vi "StomachModel.vi"() -> ()   [LabVIEW 2017]
panel:
  in  "stop":bool
  out "Ring 4 Start":u32
  out "Ring 7 Start":u32
  out "Ring 6 Start":u32
  out "Ring 5 Start":u32
  out "Ring 3 Start":u32
  out "Ring 2 Start":u32
  out "Ring 1 Start":u32
  out "Ring 0 Start":u32
  out "Run Time":u32
  in  "Time Delay 2":u32
  in  "Time Delay 1":u32
  in  "Time Delay 0":u32
  out "Ring 7":bool
  out "Ring 6":bool
  out "Ring 5":bool
  out "Ring 4":bool
  out "Ring 3":bool
  out "Ring 2":bool
  out "Ring 1":bool
  out "Time":u32
  in  "Slow Wave Generator":bool
  out "Ring 0":bool
  # "Pacemaker"
  # "Stomach Model"
  # "Ring 0"
  # "Ring 1"
  # "Ring 2"
  # "Ring 3"
  # "Ring 4"
  # "Ring 5"
  # "Corpus"
  # "Ring 6"
  # "Ring 7"
  # "Antrum"
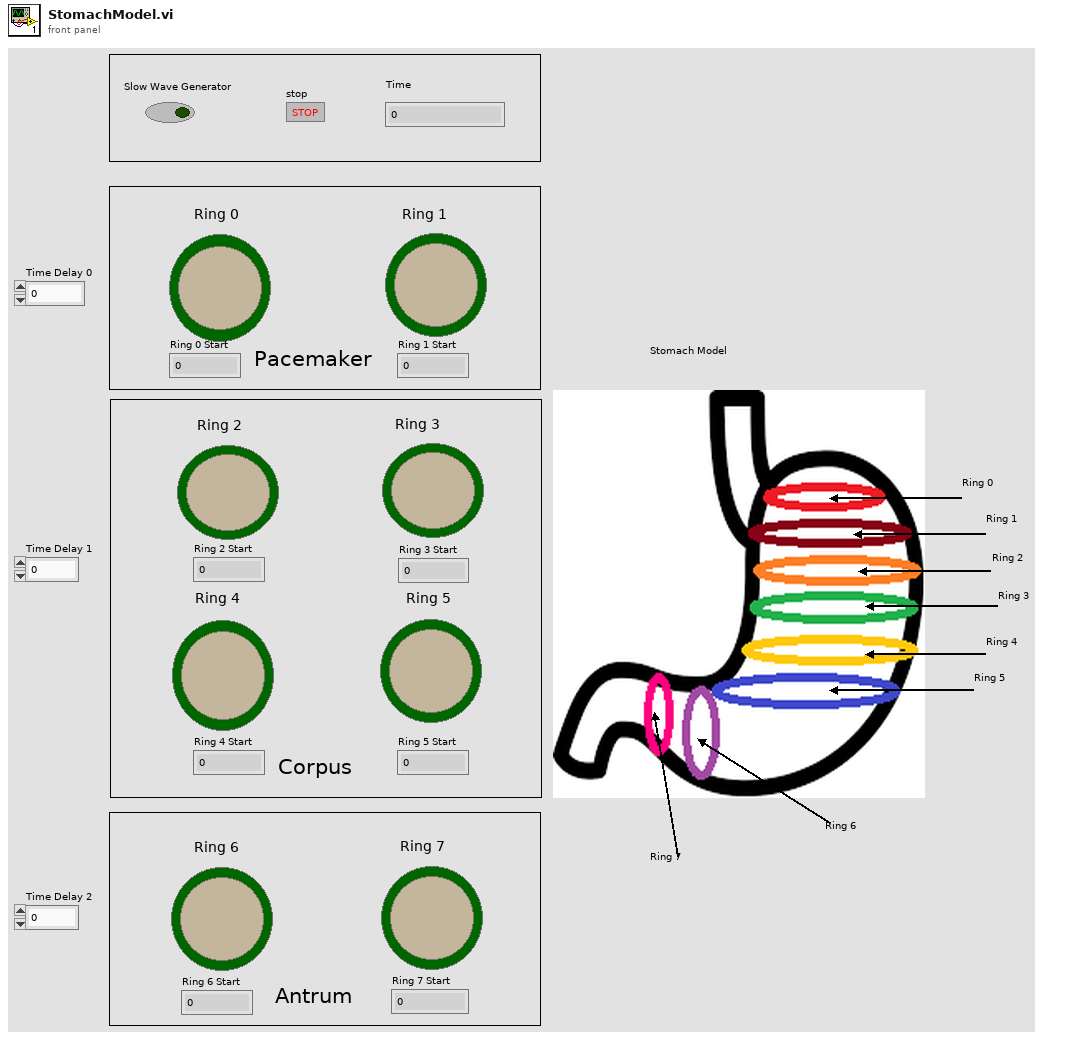
[diagram p1: front panel]
types:
  T1 = enum16{"Ring 0", "Ring 1", "Ring 2", "Ring 3", "Ring 4", "Ring 5", "Ring 6", "Ring 7"}
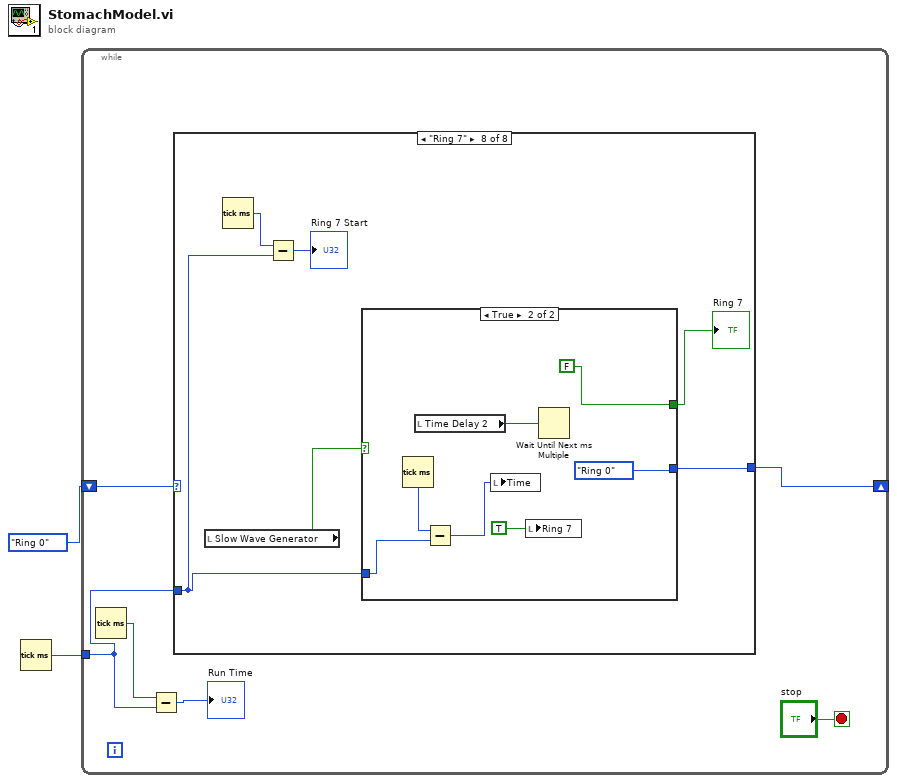
[diagram p0: block diagram]
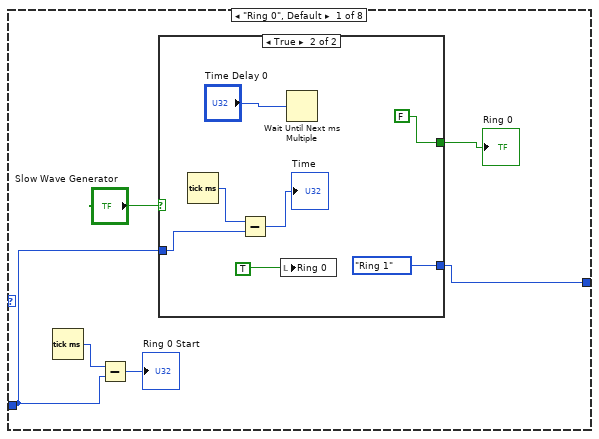
[diagram p2: hidden frame]
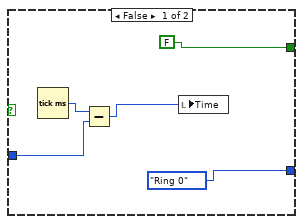
[diagram p3: hidden frame]
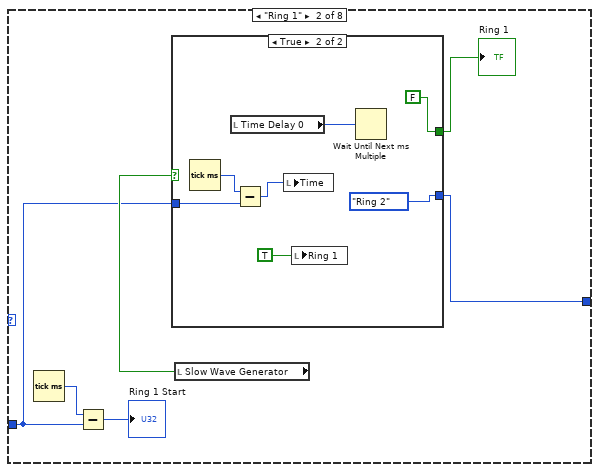
[diagram p4: hidden frame]
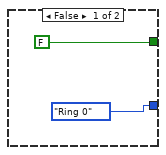
[diagram p5: hidden frame]
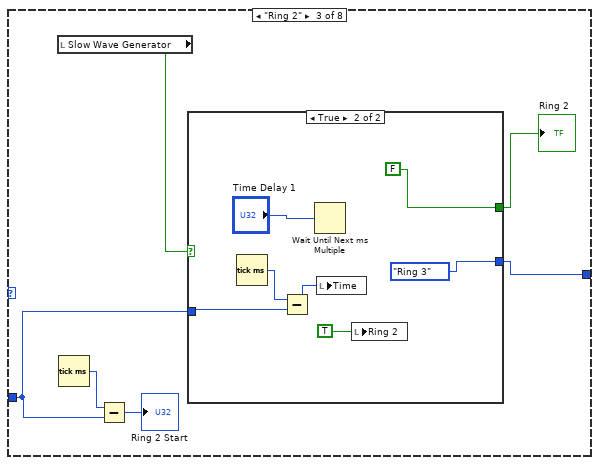
[diagram p6: hidden frame]
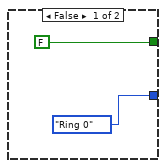
[diagram p7: hidden frame]
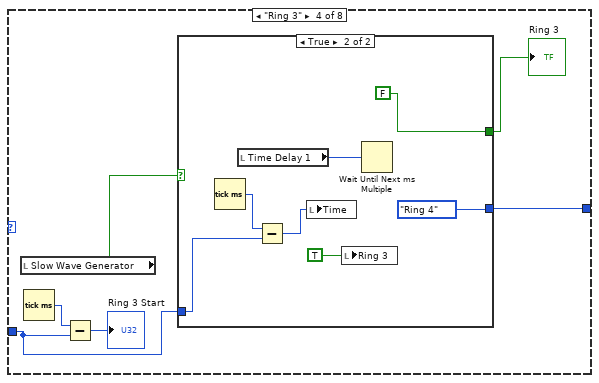
[diagram p8: hidden frame]
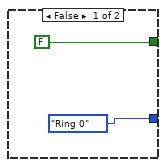
[diagram p9: hidden frame]
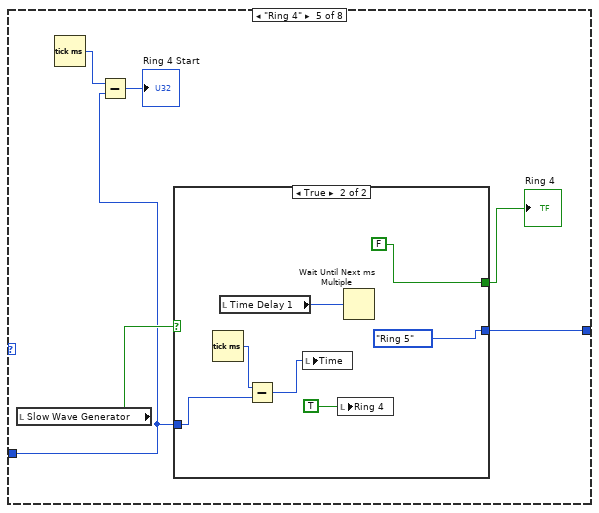
[diagram p10: hidden frame]
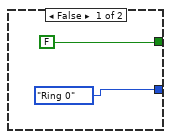
[diagram p11: hidden frame]
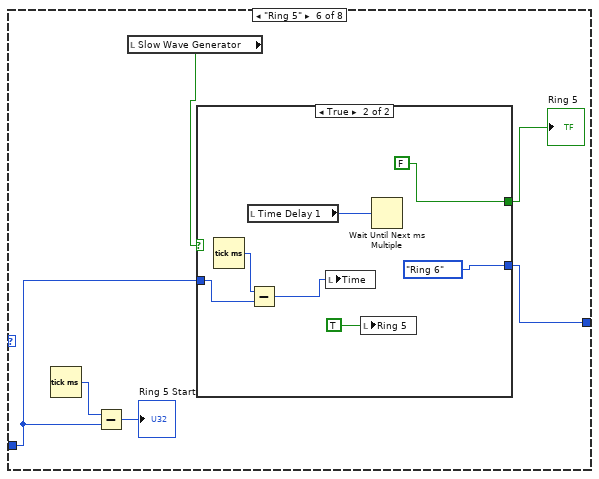
[diagram p12: hidden frame]
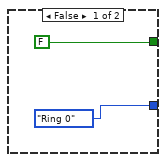
[diagram p13: hidden frame]
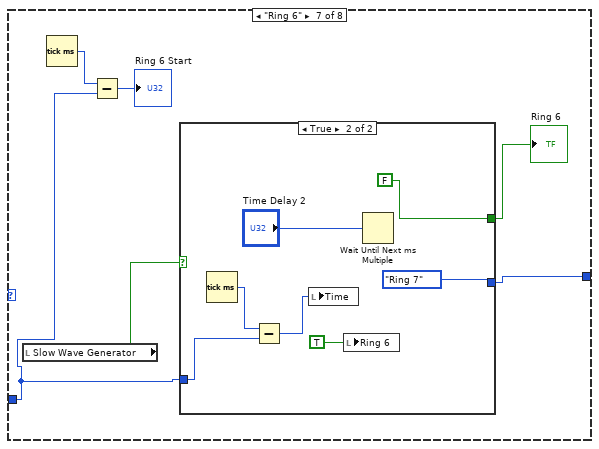
[diagram p14: hidden frame]
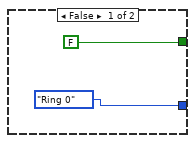
[diagram p15: hidden frame]
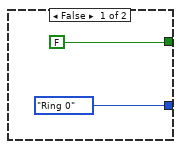
[diagram p16: hidden frame]
diagram:
  n1 = Tick Count (ms)() -> (millisecond timer value=w1:u32)
  n2 = while {
    shift-right: [w7] -> _
    shift-left: T1."Ring 0" ("Enum") -> [w8]
    tunnel: w1 -> [w4]
    stop <- "stop" stop-if-true
    n3 = Tick Count (ms)() -> (millisecond timer value=w6:u32)
    n4 = Subtract(x=w6, y=w4) -> (x-y=→"Run Time":u32)
    n5 = case shown="\"Ring 7\"" w8 {
      tunnel: [w12 w31 w45 w60 w75 w91 w105 w120] -> w7
      tunnel: w4 -> [w10 w28 w42 w57 w72 w87 w102 w117]
      frame "Ring 0", Default {
        n6 = Tick Count (ms)() -> (millisecond timer value=w11:u32)
        n7 = Subtract(x=w11, y=w10) -> (x-y=→"Ring 0 Start":u32)
        n8 = case shown="True" "Slow Wave Generator" {
          tunnel: [FALSE FALSE] -> w14
          tunnel: [T1."Ring 0" ("Enum") T1."Ring 1" ("Enum")] -> w12
          tunnel: w10 -> [w16 w21]
          frame False {
            n9 = Tick Count (ms)() -> (millisecond timer value=w17:u32)
            n10 = Subtract(x=w17, y=w16) -> (x-y=w15:u32)
            n11 = local write "Time"(w15) -> ()
          }
          frame True {
            n12 = Tick Count (ms)() -> (millisecond timer value=w22:u32)
            n13 = Subtract(x=w22, y=w21) -> (x-y=→"Time":u32)
            n14 = local write "Ring 0"(TRUE) -> ()
            n15 = Wait Until Next ms Multiple(millisecond multiple="Time Delay 0") -> ()  [unwired: 1 out]
          }
        }
        "Ring 0" <- w14
      }
      frame "Ring 1" {
        n16 = Tick Count (ms)() -> (millisecond timer value=w27:u32)
        n17 = Subtract(x=w27, y=w28) -> (x-y=→"Ring 1 Start":u32)
        n18 = local read "Slow Wave Generator"() -> (w30:bool)
        n19 = case shown="True" w30 {
          tunnel: [T1."Ring 0" ("Enum") T1."Ring 2" ("Enum")] -> w31
          tunnel: [FALSE FALSE] -> w32
          tunnel: w28 -> [_ w36]
          frame False {
          }
          frame True {
            n20 = Tick Count (ms)() -> (millisecond timer value=w37:u32)
            n21 = local read "Time Delay 0"() -> (w38:u32)
            n22 = Subtract(x=w37, y=w36) -> (x-y=w35:u32)
            n23 = local write "Time"(w35) -> ()
            n24 = local write "Ring 1"(TRUE ("Boolean 2")) -> ()
            n25 = Wait Until Next ms Multiple(millisecond multiple=w38) -> ()  [unwired: 1 out]
          }
        }
        "Ring 1" <- w32
      }
      frame "Ring 2" {
        n26 = local read "Slow Wave Generator"() -> (w46:bool)
        n27 = Tick Count (ms)() -> (millisecond timer value=w44:u32)
        n28 = Subtract(x=w44, y=w42) -> (x-y=→"Ring 2 Start":u32)
        n29 = case shown="True" w46 {
          tunnel: [FALSE FALSE] -> w47
          tunnel: [T1."Ring 0" ("Enum") T1."Ring 3" ("Enum")] -> w45
          tunnel: w42 -> [_ w50]
          frame False {
          }
          frame True {
            n30 = Tick Count (ms)() -> (millisecond timer value=w51:u32)
            n31 = Subtract(x=w51, y=w50) -> (x-y=w52:u32)
            n32 = Wait Until Next ms Multiple(millisecond multiple="Time Delay 1") -> ()  [unwired: 1 out]
            n33 = local write "Time"(w52) -> ()
            n34 = local write "Ring 2"(TRUE ("Boolean 2")) -> ()
          }
        }
        "Ring 2" <- w47
      }
      frame "Ring 3" {
        n35 = local read "Slow Wave Generator"() -> (w61:bool)
        n36 = Tick Count (ms)() -> (millisecond timer value=w59:u32)
        n37 = Subtract(x=w59, y=w57) -> (x-y=→"Ring 3 Start":u32)
        n38 = case shown="True" w61 {
          tunnel: [FALSE FALSE] -> w62
          tunnel: [T1."Ring 0" ("Enum") T1."Ring 4" ("Enum")] -> w60
          tunnel: w57 -> [_ w65]
          frame False {
          }
          frame True {
            n39 = Tick Count (ms)() -> (millisecond timer value=w67:u32)
            n40 = local read "Time Delay 1"() -> (w68:u32)
            n41 = Subtract(x=w67, y=w65) -> (x-y=w66:u32)
            n42 = local write "Time"(w66) -> ()
            n43 = local write "Ring 3"(TRUE ("Boolean 2")) -> ()
            n44 = Wait Until Next ms Multiple(millisecond multiple=w68) -> ()  [unwired: 1 out]
          }
        }
        "Ring 3" <- w62
      }
      frame "Ring 4" {
        n45 = local read "Slow Wave Generator"() -> (w76:bool)
        n46 = Tick Count (ms)() -> (millisecond timer value=w74:u32)
        n47 = Subtract(x=w74, y=w72) -> (x-y=→"Ring 4 Start":u32)
        n48 = case shown="True" w76 {
          tunnel: [FALSE FALSE] -> w77
          tunnel: [T1."Ring 0" ("Enum") T1."Ring 5" ("Enum")] -> w75
          tunnel: w72 -> [_ w81]
          frame False {
          }
          frame True {
            n49 = Tick Count (ms)() -> (millisecond timer value=w82:u32)
            n50 = local read "Time Delay 1"() -> (w83:u32)
            n51 = Subtract(x=w82, y=w81) -> (x-y=w80:u32)
            n52 = local write "Time"(w80) -> ()
            n53 = local write "Ring 4"(TRUE ("Boolean 2")) -> ()
            n54 = Wait Until Next ms Multiple(millisecond multiple=w83) -> ()  [unwired: 1 out]
          }
        }
        "Ring 4" <- w77
      }
      frame "Ring 5" {
        n55 = Tick Count (ms)() -> (millisecond timer value=w89:u32)
        n56 = Subtract(x=w89, y=w87) -> (x-y=→"Ring 5 Start":u32)
        n57 = local read "Slow Wave Generator"() -> (w90:bool)
        n58 = case shown="True" w90 {
          tunnel: [T1."Ring 0" ("Enum") T1."Ring 6" ("Enum")] -> w91
          tunnel: [FALSE FALSE] -> w92
          tunnel: w87 -> [_ w96]
          frame False {
          }
          frame True {
            n59 = Tick Count (ms)() -> (millisecond timer value=w97:u32)
            n60 = local read "Time Delay 1"() -> (w98:u32)
            n61 = Subtract(x=w97, y=w96) -> (x-y=w95:u32)
            n62 = local write "Time"(w95) -> ()
            n63 = local write "Ring 5"(TRUE ("Boolean 2")) -> ()
            n64 = Wait Until Next ms Multiple(millisecond multiple=w98) -> ()  [unwired: 1 out]
          }
        }
        "Ring 5" <- w92
      }
      frame "Ring 6" {
        n65 = local read "Slow Wave Generator"() -> (w106:bool)
        n66 = Tick Count (ms)() -> (millisecond timer value=w104:u32)
        n67 = Subtract(x=w104, y=w102) -> (x-y=→"Ring 6 Start":u32)
        n68 = case shown="True" w106 {
          tunnel: [T1."Ring 0" ("Enum") T1."Ring 7" ("Enum")] -> w105
          tunnel: [FALSE FALSE] -> w107
          tunnel: w102 -> [_ w111]
          frame False {
          }
          frame True {
            n69 = Tick Count (ms)() -> (millisecond timer value=w112:u32)
            n70 = Subtract(x=w112, y=w111) -> (x-y=w110:u32)
            n71 = local write "Time"(w110) -> ()
            n72 = local write "Ring 6"(TRUE ("Boolean 2")) -> ()
            n73 = Wait Until Next ms Multiple(millisecond multiple="Time Delay 2") -> ()  [unwired: 1 out]
          }
        }
        "Ring 6" <- w107
      }
      frame "Ring 7" {
        n74 = local read "Slow Wave Generator"() -> (w121:bool)
        n75 = Tick Count (ms)() -> (millisecond timer value=w119:u32)
        n76 = Subtract(x=w119, y=w117) -> (x-y=→"Ring 7 Start":u32)
        n77 = case shown="True" w121 {
          tunnel: [FALSE FALSE] -> w122
          tunnel: [T1."Ring 0" ("Enum") T1."Ring 0" ("Enum")] -> w120
          tunnel: w117 -> [_ w127]
          frame False {
          }
          frame True {
            n78 = Tick Count (ms)() -> (millisecond timer value=w126:u32)
            n79 = local read "Time Delay 2"() -> (w128:u32)
            n80 = Subtract(x=w126, y=w127) -> (x-y=w125:u32)
            n81 = local write "Time"(w125) -> ()
            n82 = local write "Ring 7"(TRUE ("Boolean 2")) -> ()
            n83 = Wait Until Next ms Multiple(millisecond multiple=w128) -> ()  [unwired: 1 out]
          }
        }
        "Ring 7" <- w122
      }
    }
  }
